vi "Main.vi"(11 "Module Admin":refnum<class "Delacor_lib_QMH_Cloneable Module Admin.lvclass">) -> ()   [LabVIEW 2021, in "DQMH_byOOPRef.lvlib"]
doc: "This template is based off of the Queued Message Handler design pattern and the Queued Message Handler project template that ships with LabVIEW.\n\nThe main difference is that the queue is private to this module and communication between modules is performed via Broadcast and Request events.\n\nRequest events are wrapped in public API methods and are handled in the Event Handling Loop (EHL) of this VI. Any module can register for Broadcast events sent by this module. The EHL generates messages based on user interface actions.\n\nThe Message Handling Loop (MHL) processes messages generated by the EHL, or by other messages. The messages are string values, so new messages can be added easily to the Message Cases case structure in the MHL. Each message cluster can also provide an optional value for Message Data, which is a variant that can be converted to whatever message-specific data is required.\n_____\nBased on DQMH Project Template 7.0.0.1280."
uses:
  DQMH_byOOPRef.lvlib
  <vilib>/Delacor/Delacor QMH/Libraries/Message Queue_class/Delacor_lib_QMH_Message Queue.lvclass
  <vilib>/Utility/miscctls.llb/LVPointTypeDef.ctl
  <vilib>/Delacor/Delacor QMH/Libraries/Message Queue_class/Delacor_lib_QMH_Enqueue Message (Single).vi
  Stop Argument--cluster.ctl
  <vilib>/Delacor/Delacor QMH/Libraries/Cloneable Module Admin_class/Delacor_lib_QMH_Cloneable Module Admin.lvclass
  Custom/SerDes/OOPbyRef.lvclass
  High (Reply Payload)--cluster.ctl
  High Argument--cluster.ctl
  <vilib>/ErrorRing/Error Ring.xnode
panel:
  in  "Low Update":bool
  in  "High Update":bool
  in  "Low":string
  out "Arr":string[](array[string])
  in  "High":string
  out "error out":errorcluster
  out "Status":string
  in  "Simulate EHL Error":bool
  in  "Simulate MHL Error":bool
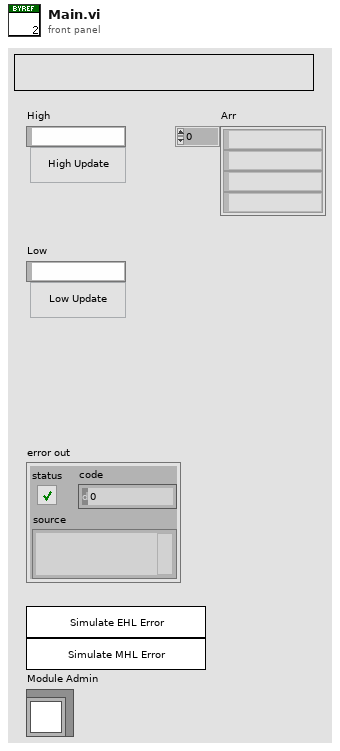
[diagram p1: front panel]
types:
  T1 = typedef "DQMH_byOOPRef.lvlib/Request Events--cluster.ctl" = cluster{"Stop Module":refnum<user-event>, "Show Panel":refnum<user-event>, "Hide Panel":refnum<user-event>, "Show Diagram":refnum<user-event>, "Get Module Execution Status":refnum<user-event>, "High":refnum<user-event>, "Low":refnum<user-event>}
  T2 = enum32{"invalid lock state", "Not Locked", "Locked (No Password)", "Password-protected"}
  T3 = typedef "DQMH_byOOPRef.lvlib/Stop Argument--cluster.ctl" = cluster{"Module ID":i32, "Origin":string, "Exit via Stop Module Req?":bool, "Wait for Module to stop?":bool}
  T4 = typedef "DQMH_byOOPRef.lvlib/High Argument--cluster.ctl" = cluster{"Module ID":i32, "Input High":string, "Wait Notifier":refnum<notifier>, "wait for reply":bool}
  T5 = typedef "LVPointTypeDef.ctl" = cluster{"Horizontal":i16, "Vertical":i16}
  T6 = enum32{"Invalid", "Standard", "Closed", "Hidden", "Minimized", "Maximized"}
  T7 = typedef "DQMH_byOOPRef.lvlib/High (Reply Payload)--cluster.ctl" = cluster{"Module ID":i32, "error":errorcluster}
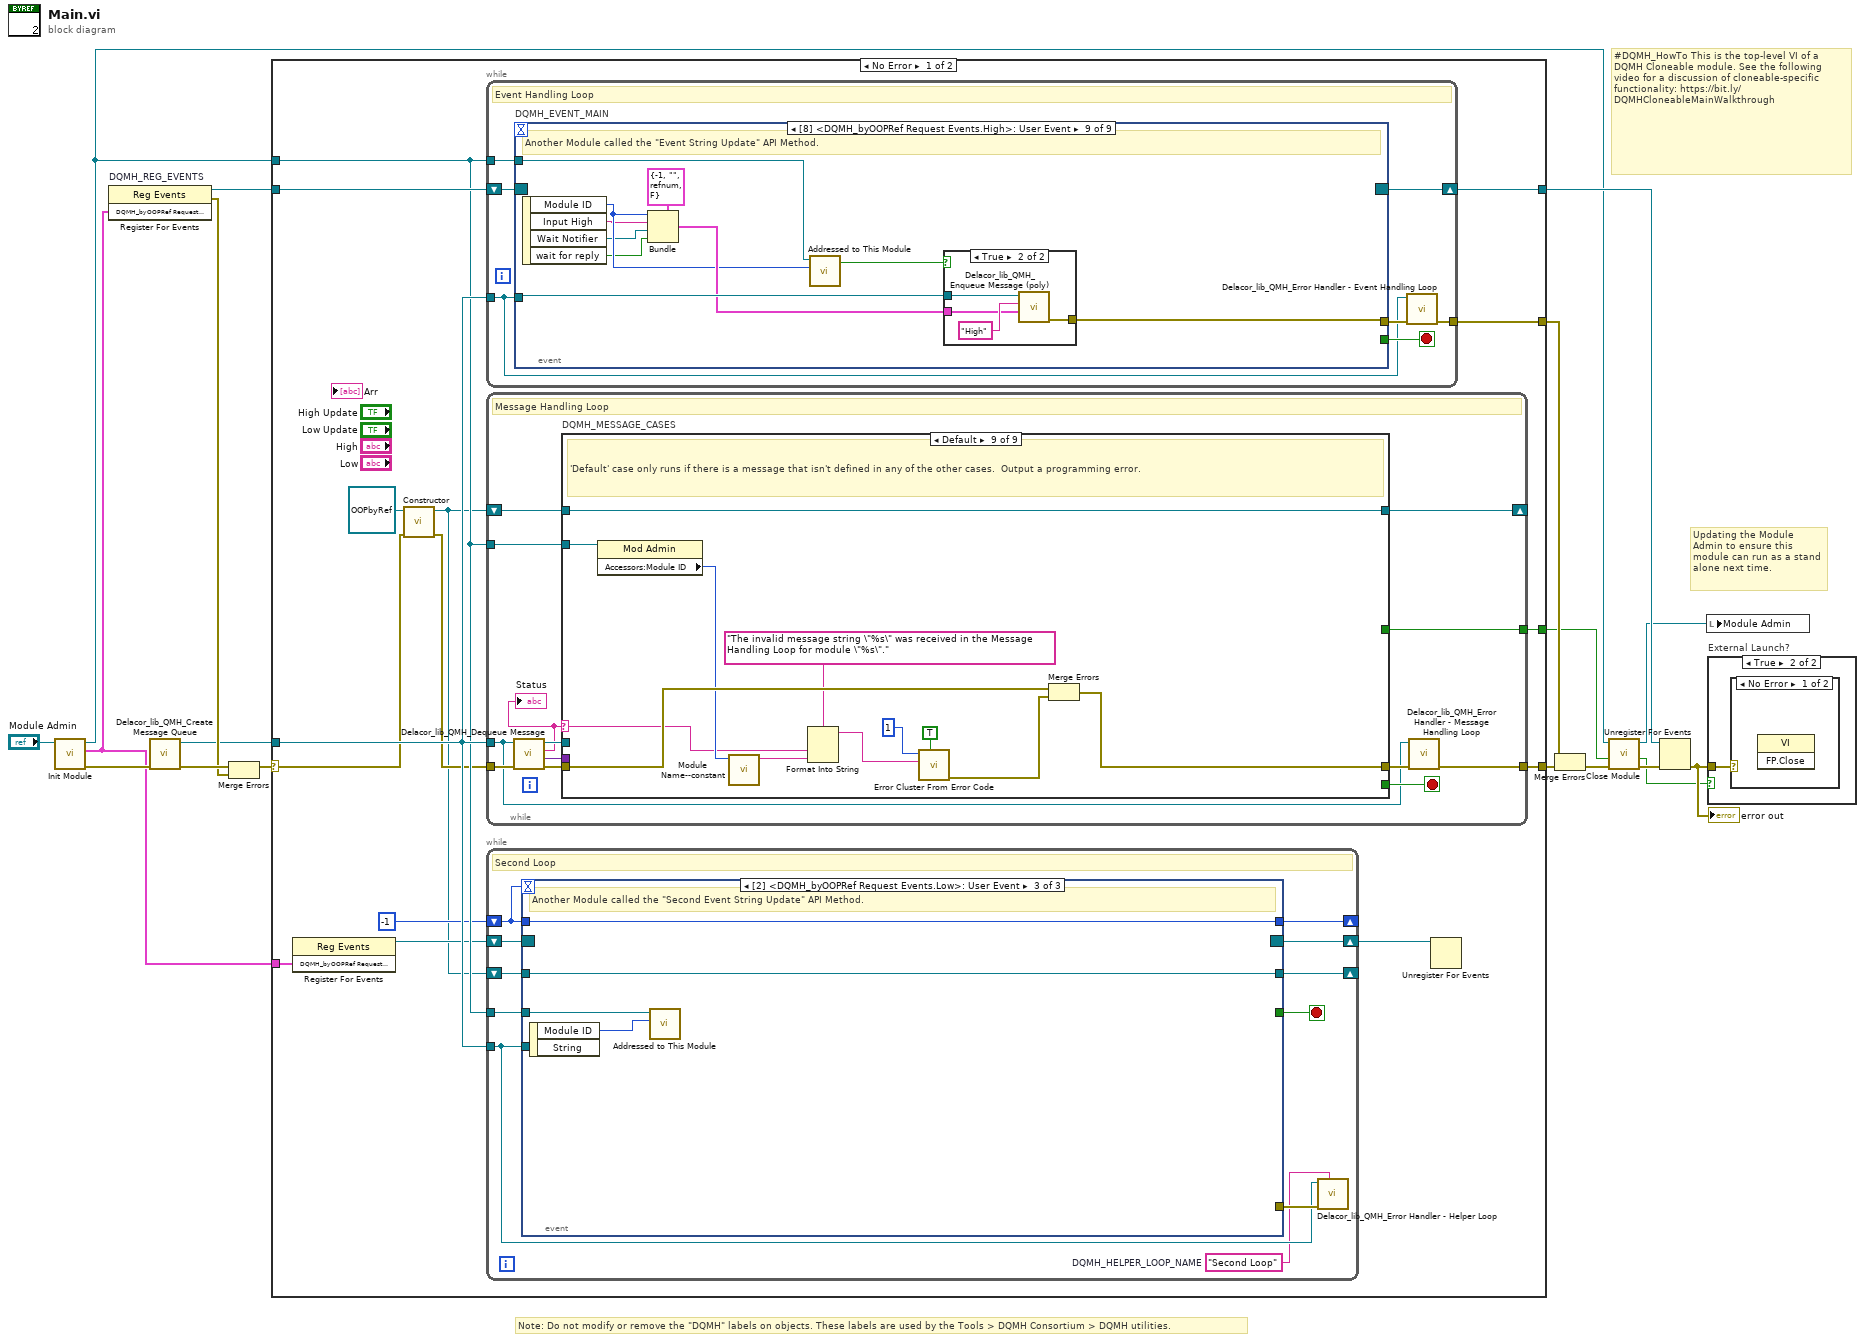
[diagram p0: block diagram]
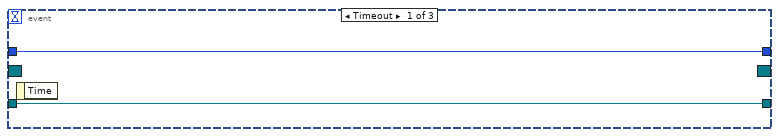
[diagram p2: hidden frame]
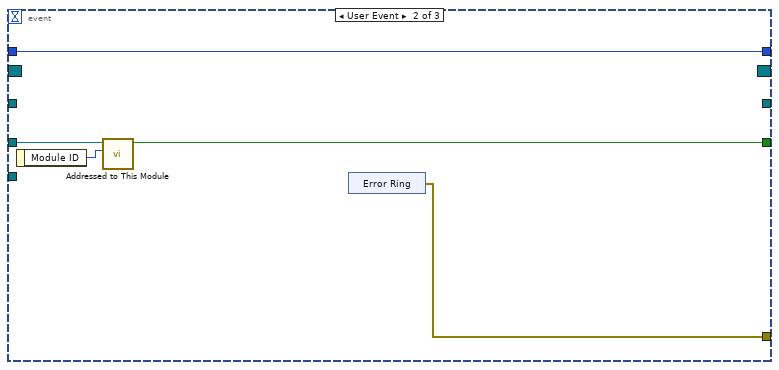
[diagram p3: hidden frame]
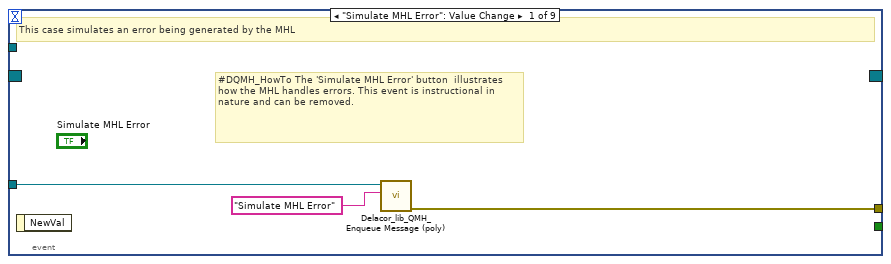
[diagram p4: hidden frame]
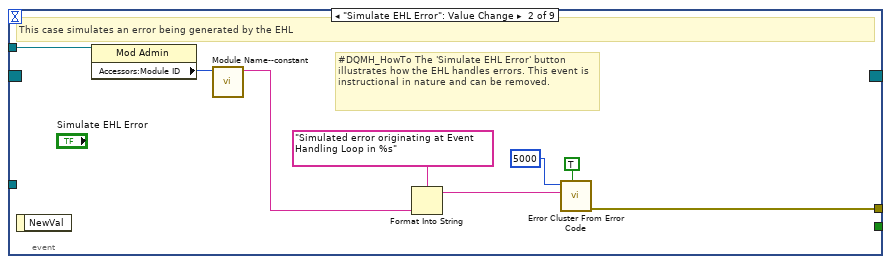
[diagram p5: hidden frame]
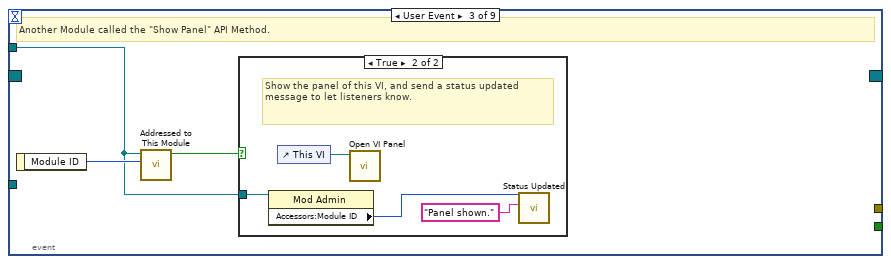
[diagram p6: hidden frame]
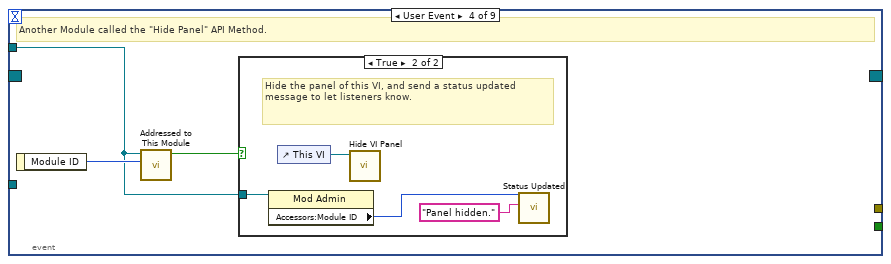
[diagram p8: hidden frame]
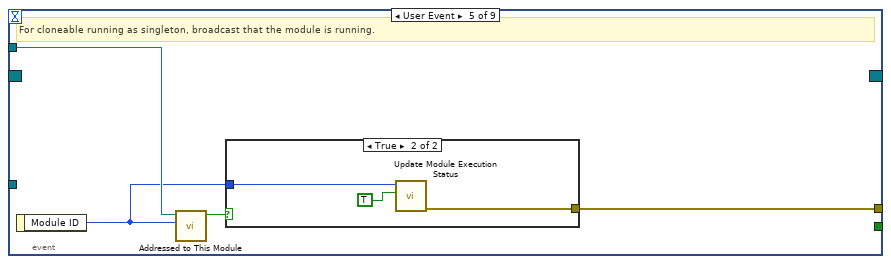
[diagram p10: hidden frame]
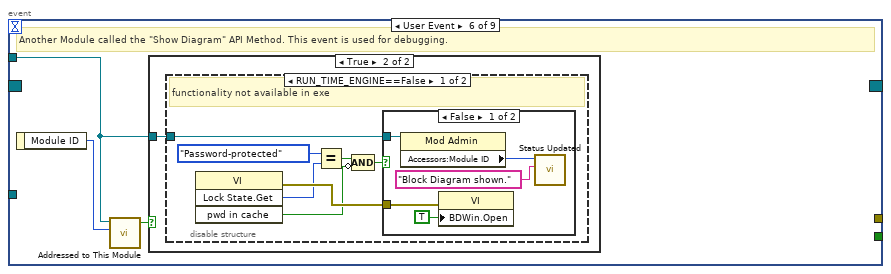
[diagram p12: hidden frame]
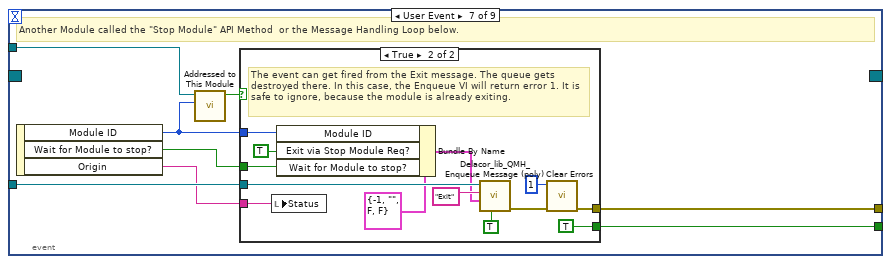
[diagram p16: hidden frame]
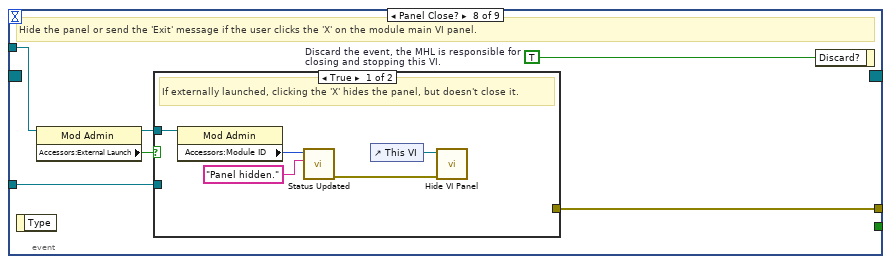
[diagram p18: hidden frame]
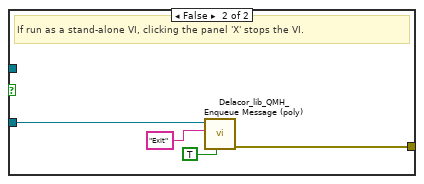
[diagram p19: hidden frame]
diagram:
  # "#DQMH_HowTo This is the top-level VI of a DQMH Cloneable module. See the following video for a discussion of cloneable-specific functionality: https://bit.ly/DQMHCloneableMainWalkthrough"
  # "Note: Do not modify or remove the \"DQMH\" labels on objects. These labels are used by the Tools > DQMH Consortium > DQMH utilities."
  # "Updating the Module Admin to ensure this module can run as a stand alone next time."
  n1 = call "Init Module.vi"("Cloneable Module Admin in"="Module Admin") -> ("error out"=w15:errorcluster, "DQMH_byOOPRef Request Events"=w1:T1, "Cloneable Module Admin out"=w5:refnum<class "Delacor_lib_QMH_Cloneable Module Admin.lvclass">)  [unwired: 8 in]
  n2 = register-events "DQMH_REG_EVENTS"(w1) -> (reference out=w8:refnum<event-registration>, error out=w10:errorcluster)  [unwired: 2 in]
  n3 = call <vilib>:"Delacor_lib_QMH_Create Message Queue.vi"("error in"=w15) -> ("error out"=w12:errorcluster, "Message Queue"=w7:refnum<class "Delacor_lib_QMH_Message Queue.lvclass">)  [unwired: 9 in]
  n4 = Merge Errors(w12, w10) -> (w11:errorcluster)
  n5 = case shown="No Error" w11 {
    selector: w11 -> [w21 w296]
    tunnel: [w33 w295] -> w16
    tunnel: [w31 w294] -> w9
    tunnel: w8 -> [w30 w294]
    tunnel: w7 -> [w29 w287]
    tunnel: [w32 _] -> w17
    tunnel: w5 -> [w28 w290]
    tunnel: [w27 _] -> w3
    tunnel: w1 -> [w26 _]
    frame No Error {
      n6 = register-events ("DQMH_HELPER_REGFOREVENTS")(w26) -> (reference out=w24:refnum<event-registration>)  [unwired: 2 in, 1 out]
      n7 = call "Constructor.vi"("error in (no error)"=w21, "SerDes in"=refnum<class "OOPbyRef.lvclass"> refnum ("Data Cluster")) -> ("error out"=w20:errorcluster, "SerDes out"=w19:refnum<class "OOPbyRef.lvclass">)  [unwired: 8 in]
      n8 = while {
        tunnel: w29 -> [w57]
        shift-right: [w60] -> w31
        shift-left: w30 -> [w61]
        tunnel: [w62] -> w32
        tunnel: w28 -> [w58]
        stop <- w59 stop-if-true
        # "Event Handling Loop"
        n9 = event "DQMH_EVENT_MAIN" shown="[8] <DQMH_byOOPRef Request Events.High>: User Event" {
          selector: w61 -> [_ _ _ _ _ _ _ _ _]
          dyn-events: [_ _ _ _ _ _ _ _ _] -> w60
          timeout: _ -> [_ _ _ _ _ _ _ _ _]
          tunnel: [_ _ _ _ _ _ w115 _ _] -> w59
          tunnel: w57 -> [w65 _ _ _ _ _ w118 w135 w157]
          tunnel: [w66 w74 _ _ w92 _ w119 w138 w148] -> w63
          tunnel: w58 -> [_ w73 w75 w82 w90 w96 w117 w136 w155]
          event "Simulate MHL Error": Value Change {
            # "#DQMH_HowTo The 'Simulate MHL Error' button  illustrates how the MHL handles errors. This event is instructional in nature and can be removed."
            # "This case simulates an error being generated by the MHL"
            n10 = event-data() -> ()  [unwired: 1 in, 1 out]
            n11 = call-poly <vilib>:"Delacor_lib_QMH_Enqueue Message (poly).vi"("Message"="Simulate MHL Error", "Message Queue in"=w65) -> ("error out"=w66:errorcluster)  [unwired: 8 in, 1 out]
          }
          event "Simulate EHL Error": Value Change {
            # "#DQMH_HowTo The 'Simulate EHL Error' button  illustrates how the EHL handles errors. This event is instructional in nature and can be removed."
            # "This case simulates an error being generated by the EHL"
            n12 = event-data() -> ()  [unwired: 1 in, 1 out]
            n13 = property class="Mod Admin"(reference=w73) -> ("Accessors:Module ID"=w72:i32)  [unwired: 1 in, 2 out]
            n14 = call "Module Name--constant.vi"("Module ID"=w72) -> ("Module Name"=w67:string)  [unwired: 10 in]
            n15 = Format Into String(format string="Simulated error originating at Event Handling Loop in %s", w67) -> (resulting string=w70:string)  [unwired: 2 in, 1 out]
            n16 = call <vilib>:"Error Cluster From Error Code.vi"("show call chain? (False)"=TRUE, "error message (\"\")"=w70, "error code (0)"=5000) -> ("error out"=w74:errorcluster)  [unwired: 6 in]
          }
          event User Event {
            # "Another Module called the \"Show Panel\" API Method."
            n17 = event-data() -> ("Module ID"=w76:i32)  [unwired: 1 in]
            n18 = call "Addressed to This Module.vi"("Module ID from Argument"=w76, "Module Admin"=w75) -> ("Addressed to this instance?"=w77:bool)  [unwired: 8 in, 1 out]
            n19 = case shown="True" w77 {
              tunnel: w75 -> [_ w79]
              frame False {
              }
              frame True {
                # "Show the panel of this VI, and send a status updated message to let listeners know."
                n20 = property class="Mod Admin"(reference=w79) -> ("Accessors:Module ID"=w78:i32)  [unwired: 1 in, 2 out]
                n21 = control-ref of="This VI"() -> (w81:refnum<vi>)
                n22 = call "Open VI Panel.vi"("VI"=w81) -> ()  [unwired: 10 in, 1 out]
                n23 = call "Status Updated.vi"("Status"="Panel shown." ("format string"), "Module ID"=w78) -> ()  [unwired: 9 in, 1 out]
              }
            }
          }
          event User Event {
            # "Another Module called the \"Hide Panel\" API Method."
            n24 = event-data() -> ("Module ID"=w83:i32)  [unwired: 1 in]
            n25 = call "Addressed to This Module.vi"("Module ID from Argument"=w83, "Module Admin"=w82) -> ("Addressed to this instance?"=w84:bool)  [unwired: 8 in, 1 out]
            n26 = case shown="True" w84 {
              tunnel: w82 -> [_ w86]
              frame False {
              }
              frame True {
                # "Hide the panel of this VI, and send a status updated message to let listeners know."
                n27 = property class="Mod Admin"(reference=w86) -> ("Accessors:Module ID"=w85:i32)  [unwired: 1 in, 2 out]
                n28 = control-ref of="This VI"() -> (w88:refnum<vi>)
                n29 = call "Hide VI Panel.vi"("VI"=w88) -> ()  [unwired: 10 in, 1 out]
                n30 = call "Status Updated.vi"("Status"="Panel hidden." ("format string"), "Module ID"=w85) -> ()  [unwired: 9 in, 1 out]
              }
            }
          }
          event User Event {
            # "For cloneable running as singleton, broadcast that the module is running."
            n31 = event-data() -> ("Module ID"=w89:i32)  [unwired: 1 in]
            n32 = call "Addressed to This Module.vi"("Module ID from Argument"=w89, "Module Admin"=w90) -> ("Addressed to this instance?"=w91:bool)  [unwired: 8 in, 1 out]
            n33 = case shown="True" w91 {
              tunnel: [_ w95] -> w92
              tunnel: w89 -> [_ w94]
              frame False {
              }
              frame True {
                n34 = call "Update Module Execution Status.vi"("Running?"=TRUE, "Module ID"=w94) -> ("error out"=w95:errorcluster)  [unwired: 9 in]
              }
            }
          }
          event User Event {
            # "Another Module called the \"Show Diagram\" API Method. This event is used for debugging."
            n35 = event-data() -> ("Module ID"=w97:i32)  [unwired: 1 in]
            n36 = call "Addressed to This Module.vi"("Module ID from Argument"=w97, "Module Admin"=w96) -> ("Addressed to this instance?"=w98:bool)  [unwired: 8 in, 1 out]
            n37 = case shown="True" w98 {
              tunnel: w96 -> [_ w99]
              frame False {
              }
              frame True {
                n38 = disable-structure shown="RUN_TIME_ENGINE==False" {
                  disable-tunnel: w99 -> [w100 _]
                  frame condition #0 (active) {
                    # "functionality not available in exe"
                    n39 = invoke class="VI" method="Lock State.Get"() -> (error out=w106:errorcluster, "Get Lock State"=w105:T2, "pwd in cache"=w102:bool)  [unwired: 4 in, 1 out]
                    n40 = Equal?(x=T2."Password-protected", y=w105) -> (x = y?=w103:bool)
                    n41 = Compound Arithmetic op=AND(w103, invert w102) -> (w101:bool)
                    n42 = case shown="False" w101 {
                      tunnel: w106 -> [w111 _]
                      tunnel: w100 -> [w108 _]
                      frame False {
                        n43 = property class="Mod Admin"(reference=w108) -> ("Accessors:Module ID"=w107:i32)  [unwired: 1 in, 2 out]
                        n44 = property class="VI"(error in=w111, "BDWin.Open"=TRUE ("Block Diagram Window:Open")) -> ()  [unwired: 1 in, 2 out]
                        n45 = call "Status Updated.vi"("Status"="Block Diagram shown." ("format string"), "Module ID"=w107) -> ()  [unwired: 9 in, 1 out]
                      }
                      frame True {
                        # "Password-protected VI, and the password is not in the cache. Do not show the diagram."
                      }
                    }
                  }
                  frame condition #1 {
                  }
                }
              }
            }
          }
          event User Event {
            # "Another Module called the \"Stop Module\" API Method  or the Message Handling Loop below."
            n46 = event-data() -> ("Module ID"=w113:i32, "Wait for Module to stop?"=w114:bool, "Origin"=w112:string)  [unwired: 1 in]
            n47 = call "Addressed to This Module.vi"("Module ID from Argument"=w113, "Module Admin"=w117) -> ("Addressed to this instance?"=w116:bool)  [unwired: 8 in, 1 out]
            n48 = case shown="True" w116 {
              tunnel: [_ w131] -> w119
              tunnel: w118 -> [_ w127]
              tunnel: [_ TRUE] -> w115
              tunnel: w114 -> [_ w122]
              tunnel: w113 -> [_ w124]
              tunnel: w112 -> [_ w120]
              frame False {
              }
              frame True {
                # "The event can get fired from the Exit message. The queue gets destroyed there. In this case, the Enqueue VI will return error 1. It is safe to ignore, because the module is already exiting."
                n49 = local write "Status"(w120) -> ()
                n50 = Bundle By Name(cluster=T3 {"Module ID"=-1, "Origin"="", "Exit via Stop Module Req?"=FALSE, "Wait for Module to stop?"=FALSE} ("Stop Argument"), "Module ID"=w124, "Exit via Stop Module Req?"=TRUE, "Wait for Module to stop?"=w122) -> (w121:T3)
                n51 = call-poly <vilib>:"Delacor_lib_QMH_Enqueue Message (poly).vi"("Priority Message? (F)"=TRUE, "Message Data"=w121, "Message"="Exit", "Message Queue in"=w127) -> ("error out"=w132:errorcluster)  [unwired: 6 in, 1 out]
                n52 = call <vilib>:"Clear Errors.vi"("error in (no error)"=w132, "specific error code to clear (0: all)"=1) -> ("error out"=w131:errorcluster)  [unwired: 4 in, 1 out]
              }
            }
          }
          event Panel Close? {
            w137 = TRUE  # Discard the event, the MHL is responsible for closing and stopping this VI.
            # "Hide the panel or send the 'Exit' message if the user clicks the 'X' on the module main VI panel."
            n53 = event-data() -> ()  [unwired: 1 in, 1 out]
            n54 = property class="Mod Admin"(reference=w136) -> (reference out=w133:refnum<class "Delacor_lib_QMH_Cloneable Module Admin.lvclass">, "Accessors:External Launch"=w134:bool)  [unwired: 1 in, 1 out]
            n55 = case shown="True" w134 {
              tunnel: w135 -> [_ w146]
              tunnel: [_ w147] -> w138
              tunnel: w133 -> [w141 _]
              frame True {
                # "If externally launched, clicking the 'X' hides the panel, but doesn't close it."
                n56 = property class="Mod Admin"(reference=w141) -> ("Accessors:Module ID"=w140:i32)  [unwired: 1 in, 2 out]
                n57 = call "Status Updated.vi"("Status"="Panel hidden." ("format string"), "Module ID"=w140) -> ("error out"=w139:errorcluster)  [unwired: 9 in]
                n58 = control-ref of="This VI"() -> (w143:refnum<vi>)
                n59 = call "Hide VI Panel.vi"("error in"=w139, "VI"=w143) -> ()  [unwired: 9 in, 1 out]
              }
              frame False {
                # "If run as a stand-alone VI, clicking the panel 'X' stops the VI."
                n60 = call-poly <vilib>:"Delacor_lib_QMH_Enqueue Message (poly).vi"("Priority Message? (F)"=TRUE, "Message"="Exit", "Message Queue in"=w146) -> ("error out"=w147:errorcluster)  [unwired: 7 in, 1 out]
              }
            }
            n61 = event-data("Discard?"=w137) -> ()  [unwired: 1 in, 1 out]
          }
          event User Event {
            # "Another Module called the \"Event String Update\" API Method."
            n62 = event-data() -> ("Module ID"=w152:i32, "Input High"=w151:string, "Wait Notifier"=w150:refnum<notifier>, "wait for reply"=w149:bool)  [unwired: 1 in]
            n63 = Bundle(cluster=T4 {"Module ID"=-1, "Input High"="", "Wait Notifier"=refnum, "wait for reply"=FALSE} ("Event String Update Argument"), "Module ID"=w152, "Input High"=w151, "Wait Notifier"=w150, "wait for reply"=w149) -> (w153:T4)
            n64 = call "Addressed to This Module.vi"("Module ID from Argument"=w152, "Module Admin"=w155) -> ("Addressed to this instance?"=w156:bool)  [unwired: 8 in, 1 out]
            n65 = case shown="True" w156 {
              tunnel: w157 -> [_ w161]
              tunnel: w153 -> [_ w159]
              tunnel: [_ w158] -> w148
              frame False {
              }
              frame True {
                n66 = call-poly <vilib>:"Delacor_lib_QMH_Enqueue Message (poly).vi"("Message Data"=w159, "Message"="High", "Message Queue in"=w161) -> ("error out"=w158:errorcluster)  [unwired: 7 in, 1 out]
              }
            }
          }
        }
        n67 = call-dynamic "Delacor_lib_QMH_Error Handler - Event Handling Loop.vi"("error in"=w63, "Message Queue in"=w57) -> ("dup error in"=w62:errorcluster)  [unwired: 8 in, 1 out]
      }
      n68 = while {
        tunnel: w29 -> [w163]
        shift-right: [w169] -> _
        shift-left: w19 -> [w170]
        tunnel: w20 -> [w173]
        tunnel: [w171] -> w33
        tunnel: w28 -> [w165]
        tunnel: [w164] -> w27
        stop <- w168 stop-if-true
        # "Message Handling Loop"
        n69 = call-dynamic "Delacor_lib_QMH_Dequeue Message.vi"("error in"=w173, "Message Queue in"=w163) -> ("error out"=w172:errorcluster, "Message Data"=w167:variant, "Message"=w162:string, "Message Queue out"=w166:refnum<class "Delacor_lib_QMH_Message Queue.lvclass">)  [unwired: 6 in]
        "Status" <- w162
        n70 = case "DQMH_MESSAGE_CASES" shown="Default" w162 {
          selector: w162 -> [_ _ _ _ _ _ _ _ w276]
          tunnel: w166 -> [_ _ _ _ _ w231 _ w268 _]
          tunnel: w172 -> [w191 w195 w208 w226 w228 w240 w257 w274 w285]
          tunnel: [w189 w195 w204 w225 w228 w236 w256 w269 w286] -> w174
          tunnel: w170 -> [w182 w194 w197 w224 w227 w235 w254 w267 w283]
          tunnel: [w182 w194 w198 w224 w227 w235 w254 w267 w283] -> w169
          tunnel: [_ _ _ _ _ _ _ w266 _] -> w168
          tunnel: w167 -> [_ _ w206 _ _ w234 _ w264 _]
          tunnel: w165 -> [w177 _ w200 _ _ w233 w252 w259 w282]
          tunnel: [_ _ _ _ _ _ _ w262 _] -> w164
          frame "Initialize" {
            # "Initialize - Any operation that needs to be done before the module can receive messages. Synchronize Caller Events.vi will inform Start Module.vi that the module has launched and is ready to receive messages. Module Did Init.vi will broadcast that the module initialized."
            n71 = call "Synchronize Caller Events.vi"("error in"=w191, "Module Admin"=w177) -> ("error out"=w190:errorcluster, "Module Admin out"=w176:refnum<class "Delacor_lib_QMH_Cloneable Module Admin.lvclass">)  [unwired: 8 in]
            n72 = property class="Mod Admin"(reference=w176) -> ("Accessors:Module ID"=w179:i32, "Accessors:External Launch"=w178:bool)  [unwired: 1 in, 2 out]
            n73 = call "Module Name--constant.vi"("Module ID"=w179) -> ("Module Name"=w186:string)  [unwired: 10 in]
            n74 = property class="VI"("Front Panel.Title"=w186) -> (reference out=w188:refnum<vi>, error out=w193:errorcluster)  [unwired: 2 in]
            n75 = Select(t=T6."Hidden" ("State"), s=w178, f=T6."Standard" ("State")) -> (s? t:f=w183:T6)
            n76 = invoke class="VI" method="FP.Open"(reference=w188, error in=w193, "State"=w183) -> (reference out=w187:refnum<vi>, error out=w192:errorcluster)  [unwired: 2 in, 3 out]
            n77 = call "Module Name--constant.vi"("Module ID"=w179) -> ("Module Name"=w180:string)  [unwired: 10 in]
            n78 = invoke class="VI" method="FP.Center"(reference=w187, error in=w192) -> ()  [unwired: 1 in, 3 out]
            n79 = call "Module Did Init.vi"("error in"=w190, "Initialized?"=TRUE, "Origin"=w180, "Module ID"=w179) -> ("error out"=w189:errorcluster)  [unwired: 7 in]
            n80 = property on="Pane" class="Pane"("Origin"=T5 {"Horizontal"=0, "Vertical"=0}) -> ()  [unwired: 2 in, 2 out]
          }
          frame "---Module Specific---" {
            # "Separator -- The following cases handle messages specific to this Module."
          }
          frame "High" {
            n81 = Variant To Data(error in=w208, type=T4 {"Module ID"=-1, "Input High"="", "Wait Notifier"=refnum, "wait for reply"=FALSE} ("Event String Update Argument"), Variant=w206) -> (data=w202:T4, error out=w207:errorcluster)
            n82 = Unbundle By Name(w202) -> ("Module ID"=w201:i32)
            n83 = property class="Mod Admin"(reference=w200) -> ("Accessors:Module ID"=w203:i32)  [unwired: 1 in, 2 out]
            n84 = call "Addressed to This Module.vi"("Module ID from Argument"=w201, "Module Admin"=w200) -> ("Addressed to this instance?"=w199:bool)  [unwired: 8 in, 1 out]
            n85 = case shown="True" w199 {
              tunnel: w203 -> [_ w217]
              tunnel: w202 -> [_ w216]
              tunnel: [w210 w214] -> w198
              tunnel: w197 -> [w210 w215]
              tunnel: [w209 w213] -> w196
              frame False {
                n86 = xnode "Error Ring"() -> ("error out"=w209:errorcluster)
              }
              frame True {
                n87 = Unbundle By Name(w216) -> ("Input High"=w212:string)
                n88 = call "High Update.vi"("Input High"=w212, "SerDes in"=w215) -> ("error out"=w213:errorcluster, "SerDes out"=w214:refnum<class "OOPbyRef.lvclass">)  [unwired: 8 in]
                n89 = Bundle By Name(cluster=T7 {"Module ID"=-1, "error"={"status"=FALSE, "code"=0, "source"=""}} ("Event String Update (Reply Payload)"), "Module ID"=w217, "error"=w213) -> (w219:T7)
                n90 = Unbundle By Name(w216) -> ("Wait Notifier"=w221:refnum<notifier>, "wait for reply"=w220:bool)
                n91 = case "DQMH_FIRE_NOTIFIER" shown="True" w220 {
                  tunnel: w221 -> [_ w223]
                  tunnel: w219 -> [_ w222]
                  frame False {
                  }
                  frame True {
                    n92 = Send Notification(notification=w222, notifier=w223) -> ()  [unwired: 1 in, 2 out]
                  }
                }
              }
            }
            n93 = Merge Errors(w207, w196) -> (w204:errorcluster)
          }
          frame "---Copy This Frame---" {
            # "Duplicate this frame when creating new messages.  Change this comment in the duplicated frame to describe this message."
            n94 = Merge Errors(w226) -> (w225:errorcluster)
          }
          frame "---Exit and Error Handling---" {
            # "Separator - the following cases handle errors and exit messages."
          }
          frame "Error" {
            # "#CodeRecommended - If the module is running in standalone mode (External Launch = FALSE), this code will pop up an error dialog and call the 'Exit' message if an error occurs. Add more fine-grained error management here."
            # "Error - Check the error message data and respond accordingly. This message is sent by the \"Error Handler\" VIs at the end of each loop in this application."
            n95 = property class="Mod Admin"(reference=w233) -> ("Accessors:External Launch"=w232:bool, "Accessors:Module ID"=w230:i32)  [unwired: 1 in, 2 out]
            n96 = Variant To Data(error in=w240, type=errorcluster {"status"=FALSE, "code"=0, "source"=""} ("error constant"), Variant=w234) -> (data=w229:errorcluster, error out=w238:errorcluster)
            n97 = local write "error out"(w229) -> ()
            n98 = call "Error Reported.vi"("Error"=w229, "Module ID"=w230) -> ()  [unwired: 9 in, 1 out]
            n99 = case shown="False" w232 {
              tunnel: [w245 _] -> w237
              tunnel: w231 -> [w243 _]
              tunnel: w229 -> [w244 _]
              frame False {
                n100 = disable-structure shown="Default" {
                  disable-tunnel: w244 -> [w246 _]
                  frame condition #0 (active) {
                    # "If the module is running standalone, then pop up an error dialog and call the \"Exit\" message."
                    n101 = call <vilib>:"Simple Error Handler.vi"("error in (no error)"=w246) -> ()  [unwired: 4 in, 5 out]
                  }
                  frame condition #1 {
                    # "To prevent the Simple Error Handler VI from being loaded (e.g. when deploying to a Real-Time target), add the Conditional Disable Symbol \"DQMH_Disable_SEH\" to your project and set it to TRUE."
                  }
                }
                n102 = call-poly <vilib>:"Delacor_lib_QMH_Enqueue Message (poly).vi"("Priority Message? (F)"=TRUE, "Message"="Exit", "Message Queue in"=w243) -> ("error out"=w245:errorcluster)  [unwired: 7 in, 1 out]
              }
              frame True {
                # "If the module was launched externally, calling the Error Reported broadcast VI is the only action performed by the \"Error\" message. The module's caller can then process the error appropriately."
              }
            }
            n103 = Merge Errors(w238, w237) -> (w236:errorcluster)
          }
          frame "Simulate MHL Error" {
            # "#DQMH_HowTo The 'Simulate MHL Error' button  illustrates how the MHL handles errors. This event is instructional in nature and can be removed."
            # "Simulate an error occurring at the MHL"
            n104 = property class="Mod Admin"(reference=w252) -> ("Accessors:Module ID"=w253:i32)  [unwired: 1 in, 2 out]
            n105 = call "Module Name--constant.vi"("Module ID"=w253) -> ("Module Name"=w248:string)  [unwired: 10 in]
            n106 = Format Into String(format string="Simulated error originating at Message Handling Loop in %s", w248) -> (resulting string=w249:string)  [unwired: 2 in, 1 out]
            n107 = call <vilib>:"Error Cluster From Error Code.vi"("show call chain? (False)"=TRUE, "error message (\"\")"=w249, "error code (0)"=5001) -> ("error out"=w255:errorcluster)  [unwired: 6 in]
            n108 = Merge Errors(w257, w255) -> (w256:errorcluster)
          }
          frame "Exit" {
            w265 = 91  # 91: not all Exit messages will have an argument
            w266 = TRUE  # Stop the VI
            # "Release the message queue reference"
            # "#CodeNeeded - Add any required cleanup code here."
            # "Exit - Exit the application."
            n109 = Variant To Data(error in=w274, type=T3 {"Module ID"=-1, "Origin"="", "Exit via Stop Module Req?"=FALSE, "Wait for Module to stop?"=FALSE} ("Stop Argument"), Variant=w264) -> (data=w261:T3, error out=w270:errorcluster)
            n110 = call <vilib>:"Clear Errors.vi"("error in (no error)"=w270, "specific error code to clear (0: all)"=w265) -> ("error out"=w273:errorcluster)  [unwired: 4 in, 1 out]
            n111 = property class="Mod Admin"(reference=w259) -> ("Accessors:Module ID"=w258:i32)  [unwired: 1 in, 2 out]
            n112 = control-ref of="This VI"() -> (w260:refnum<vi>)
            n113 = call-dynamic "Delacor_lib_QMH_Release Message Queue.vi"("error in"=w273, "Message Queue"=w268) -> ("error out"=w272:errorcluster)  [unwired: 9 in]
            n114 = call "Handle Exit.vi"("Stop Argument"=w261, "Module Admin in"=w259, "VI reference"=w260) -> ("error out"=w271:errorcluster, "Wait for Stop?"=w262:bool)  [unwired: 7 in]
            n115 = Merge Errors(w272, w271) -> (w269:errorcluster)
            n116 = call "Error Reported.vi"("Error"=w269, "Module ID"=w258) -> ()  [unwired: 9 in, 1 out]
          }
          frame Default {
            # "'Default' case only runs if there is a message that isn't defined in any of the other cases.  Output a programming error."
            n117 = property class="Mod Admin"(reference=w282) -> ("Accessors:Module ID"=w281:i32)  [unwired: 1 in, 2 out]
            n118 = call "Module Name--constant.vi"("Module ID"=w281) -> ("Module Name"=w275:string)  [unwired: 10 in]
            n119 = Format Into String(format string="The invalid message string \"%s\" was received in the Message Handling Loop for module \"%s\".", w276, w275) -> (resulting string=w278:string)  [unwired: 2 in, 1 out]
            n120 = call <vilib>:"Error Cluster From Error Code.vi"("show call chain? (False)"=TRUE, "error message (\"\")"=w278, "error code (0)"=1) -> ("error out"=w284:errorcluster)  [unwired: 6 in]
            n121 = Merge Errors(w285, w284) -> (w286:errorcluster)
          }
        }
        n122 = call-dynamic "Delacor_lib_QMH_Error Handler - Message Handling Loop.vi"("error in"=w174, "Message Queue in"=w163) -> ("dup error in"=w171:errorcluster)  [unwired: 8 in, 1 out]
      }
      n123 = while "DQMH_HELPER_LOOP" {
        shift-right: [w44] -> _
        shift-left: -1 -> [w43]
        shift-right: [w41] -> w25
        shift-left: w24 -> [w42]
        tunnel: w29 -> [w38]
        tunnel: w28 -> [w36]
        shift-right: [w34] -> _
        shift-left: w19 -> [w35]
        stop <- w40 stop-if-true
        w37 = "Second Loop"  # DQMH_HELPER_LOOP_NAME
        # "Second Loop"
        n124 = event "DQMH_HELPER_EVENT_STRUCTURE" shown="[2] <DQMH_byOOPRef Request Events.Low>: User Event" {
          selector: w42 -> [_ _ _]
          dyn-events: [_ _ _] -> w41
          timeout: w43 -> [_ _ _]
          tunnel: w43 -> [w46 w51 w54]
          tunnel: [w46 w51 w54] -> w44
          tunnel: [_ w49 _] -> w40
          tunnel: [_ w47 _] -> w39
          tunnel: w38 -> [_ _ _]
          tunnel: w36 -> [_ w50 w56]
          tunnel: w35 -> [w45 _ w53]
          tunnel: [w45 _ w53] -> w34
          event Timeout {
            n125 = event-data() -> ()  [unwired: 1 in, 1 out]
          }
          event User Event {
            n126 = event-data() -> ("Module ID"=w48:i32)  [unwired: 1 in]
            n127 = call "Addressed to This Module.vi"("Module ID from Argument"=w48, "Module Admin"=w50) -> ("Addressed to this instance?"=w49:bool)  [unwired: 8 in, 1 out]
            n128 = xnode "Error Ring"() -> ("error out"=w47:errorcluster)
          }
          event User Event {
            # "Another Module called the \"Second Event String Update\" API Method."
            n129 = event-data() -> ("Module ID"=w55:i32)  [unwired: 1 in, 1 out]
            n130 = call "Addressed to This Module.vi"("Module ID from Argument"=w55, "Module Admin"=w56) -> ()  [unwired: 8 in, 2 out]
          }
        }
        n131 = call-dynamic "Delacor_lib_QMH_Error Handler - Helper Loop.vi"("Error Debug"=w37, "error in"=w39, "Message Queue in"=w38) -> ()  [unwired: 7 in, 2 out]
      }
      n132 = Unregister For Events(event registration refnum=w25) -> ()  [unwired: 1 in, 1 out]
    }
    frame Error {
      n133 = call "Synchronize Caller Events.vi"("Module Admin"=w290) -> ("Module Admin out"=w289:refnum<class "Delacor_lib_QMH_Cloneable Module Admin.lvclass">)  [unwired: 9 in, 1 out]
      n134 = property class="Mod Admin"(reference=w289) -> ("Accessors:Module ID"=w288:i32)  [unwired: 1 in, 2 out]
      n135 = call-dynamic "Delacor_lib_QMH_Release Message Queue.vi"("error in"=w296, "Message Queue"=w287) -> ("error out"=w295:errorcluster)  [unwired: 9 in]
      n136 = call "Module Name--constant.vi"("Module ID"=w288) -> ("Module Name"=w293:string)  [unwired: 10 in]
      n137 = Format Into String(format string="An error occurred during initialization. %s is no longer running.", w293) -> (resulting string=w291:string)  [unwired: 2 in, 1 out]
      n138 = call "Error Reported.vi"("Additional Information"=w291, "Error"=w295, "Module ID"=w288) -> ()  [unwired: 8 in, 1 out]
    }
  }
  n139 = Merge Errors(w17, w16) -> (w18:errorcluster)
  n140 = call "Close Module.vi"("error in"=w18, "Wait for stop?"=w3, "Module Admin in"=w5) -> ("error out"=w14:errorcluster, "External Launch"=w2:bool, "Module Admin out"=w4:refnum<class "Delacor_lib_QMH_Cloneable Module Admin.lvclass">)  [unwired: 6 in]
  n141 = Unregister For Events(event registration refnum=w9, error in=w14) -> (error out=w13:errorcluster)
  "error out" <- w13
  n142 = local write "Module Admin"(w4) -> ()
  n143 = case "External Launch?" shown="True" w2 {
    tunnel: w13 -> [_ w297]
    frame False {
    }
    frame True {
      n144 = case shown="No Error" w297 {
        frame No Error {
          n145 = invoke class="VI" method="FP.Close"() -> ()  [unwired: 3 in, 3 out]
        }
        frame Error {
          n146 = invoke class="VI" method="FP.Open"("Activate"=TRUE ("Activate?")) -> ()  [unwired: 4 in, 5 out]
        }
      }
    }
  }
